vi "Teleop.vi"(10 "Match Info":T1={"Autonomous Elapsed Seconds"=0.0, "TeleOp Elapsed Seconds"=0.0, "Disabled Elapsed Seconds"=0.0, "Visited Autonomous"=FALSE, "Visited TeleOp"=FALSE, "Visited Disabled"=FALSE, "Autonomous Settings"={"Autonomous Style"=enum."Independent", "VI Refnum"=refnum}}, 11 "Call Context":T2) -> ()   [LabVIEW 2015]
doc: "This VI is called for each TeleOp packet received from the DS where the robot is not disabled. It is often used to read from the joysticks and update I/O or to update setpoints for timed control loops. It should complete and return within 20 milliseconds or it may miss DS packets."
uses:
  <vilib>/Rock Robotics/WPI/DriverStation/WPI_DriverStationDerivedRobotMode.ctl
  <vilib>/Rock Robotics/WPI/DriverStation/WPI_DriverStationMatch Info.ctl
  Common/Change Detect.vi
  Common/Change Detect Boolean.vi
  <vilib>/Rock Robotics/Network Tables/NT Read Boolean.vi
  <vilib>/Rock Robotics/Network Tables/NT Read Number.vi
  Robot Global Data.vi
  <vilib>/Rock Robotics/WPI/Utilities/WPI_GetSetVariantRefNum.vi
panel:
  out "Sample Slider 0":dbl(slide) scale=0.0..5.0
  out "Sample Boolean 1":bool
  out "Sample Boolean 0":bool
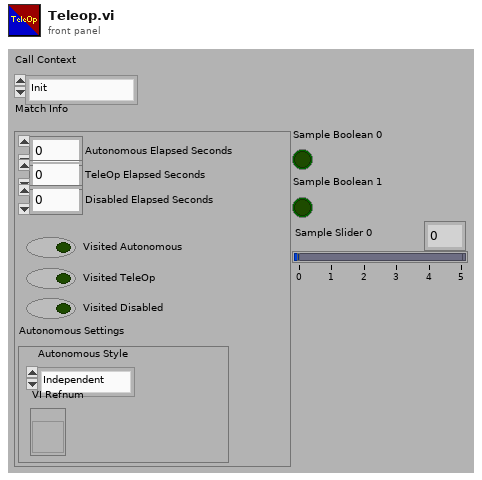
[diagram p1: front panel]
types:
  T1 = typedef "WPI_DriverStationMatch Info.ctl" = cluster{"Autonomous Elapsed Seconds":dbl, "TeleOp Elapsed Seconds":dbl, "Disabled Elapsed Seconds":dbl, "Visited Autonomous":bool, "Visited TeleOp":bool, "Visited Disabled":bool, "Autonomous Settings":cluster{"Autonomous Style":enum16{"Iterative", "Independent"}, "VI Refnum":refnum<vi>}}
  T2 = typedef "WPI_DriverStationDerivedRobotMode.ctl" = enum16{"Init", "Execute", "Stop"}
  T3 = typedef "WPI_DriverStationRobotMode2.ctl" = enum16{"Autonomous Disabled", "Autonomous Enabled", "Teleop Disabled", "Teleop Enabled", "Disconnected", "Finish", "Test Disabled", "Test Enabled", "Emergency Stopped"}
  T4 = typedef "WPI_JoystickDevRef.ctl" = cluster{"Device":T5}
  T5 = typedef "WPI_JoystickDeviceEnum.ctl" = enum16{"USB 0", "USB 1", "USB 2", "USB 3", "USB 4", "USB 5"}
  T6 = cluster{"Axes[0]":dbl, "Axes[1]":dbl, "Axes[2]":dbl, "Axes[3]":dbl, "Axes[4]":dbl, "Axes[5]":dbl, "Axes[6]":dbl, "Axes[7]":dbl, "Axes[8]":dbl}
  T7 = cluster{"Buttons[0]":bool, "Buttons[1]":bool, "Buttons[2]":bool, "Buttons[3]":bool, "Buttons[4]":bool, "Buttons[5]":bool, "Buttons[6]":bool, "Buttons[7]":bool, "Buttons[8]":bool}
  T8 = cluster{"Left_Trigger":dbl, "Right_Trigger ":dbl, "Left_X":dbl, "Left_Y":dbl, "Right_X":dbl, "Right_Y":dbl}
  T9 = cluster{"A":bool, "B":bool, "X":bool, " Y":bool, "LB":bool, " RB":bool, "Left_Thumb_Button":bool, "Right_Thumb_Button":bool, "Back":bool, "Start":bool}
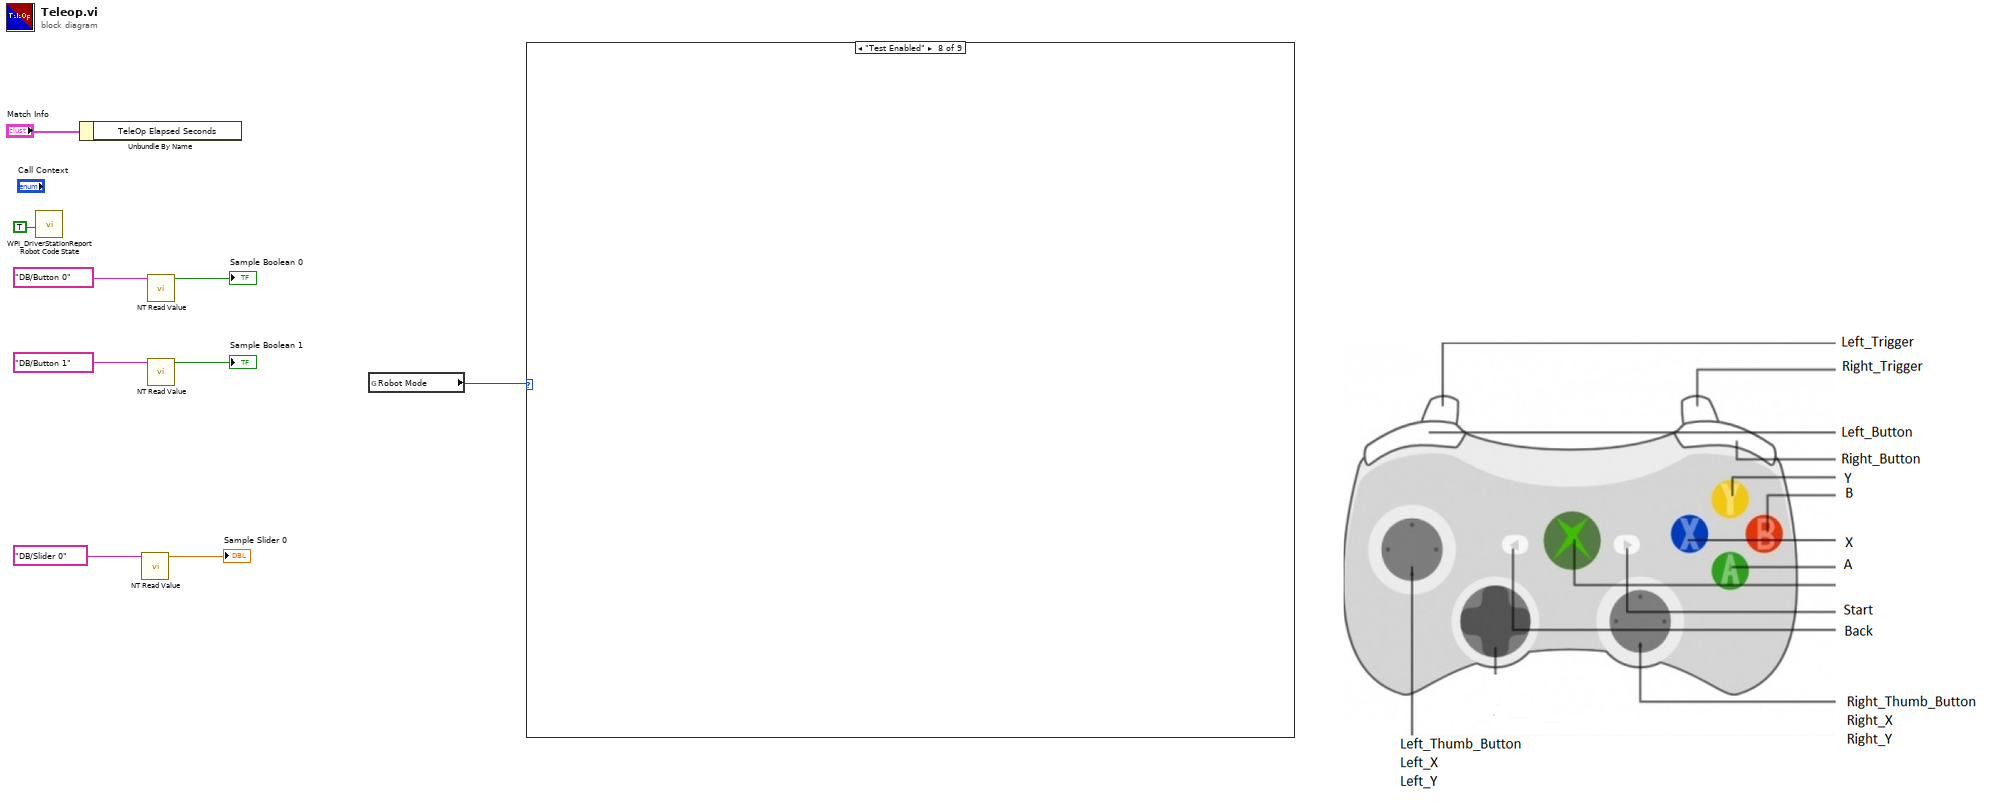
[diagram p0: block diagram]
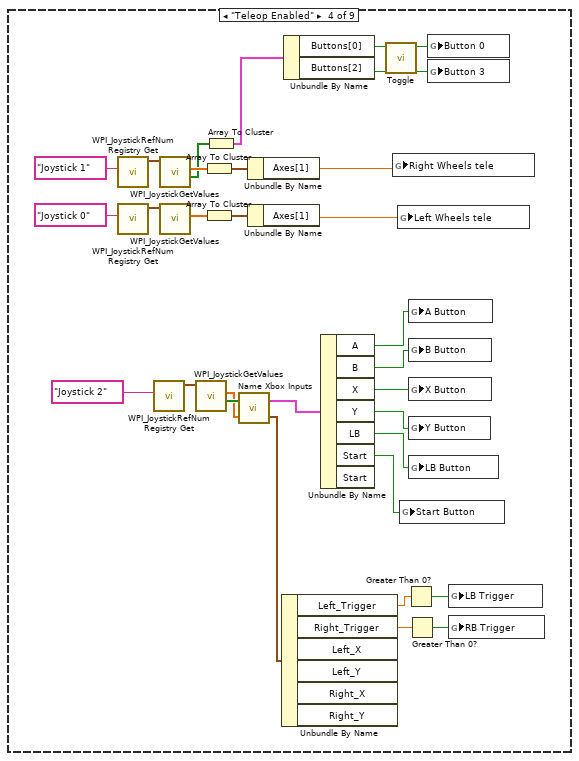
[diagram p5: hidden frame]
diagram:
  n1 = call <vilib>:"WPI_DriverStationReport Robot Code State.vi"("TeleOp"=TRUE ("Autonomous")) -> ()  [unwired: 10 in, 1 out]
  n2 = Unbundle By Name("Match Info") -> ()  [unwired: 1 out]
  n3 = call-poly <vilib>:"NT Read Value.vi"("Name"="DB/Slider 0" ("refnum name")) -> ("Numeric"=→"Sample Slider 0":dbl)  [unwired: 9 in, 1 out]
  n4 = call-poly <vilib>:"NT Read Value.vi"("Name"="DB/Button 0" ("refnum name")) -> ("Boolean"=→"Sample Boolean 0":bool)  [unwired: 9 in, 1 out]
  n5 = call-poly <vilib>:"NT Read Value.vi"("Name"="DB/Button 1" ("refnum name")) -> ("Boolean"=→"Sample Boolean 1":bool)  [unwired: 9 in, 1 out]
  n6 = global read "Robot Global Data.vi" "Robot Mode"() -> (w1:T3)
  n7 = case shown="\"Test Enabled\"" w1 {
    frame "Autonomous Disabled", Default {
    }
    frame "Autonomous Enabled" {
    }
    frame "Teleop Disabled" {
    }
    frame "Teleop Enabled" {
      n8 = call <vilib>:"WPI_JoystickRefNum Registry Get.vi"("refnum name"="Joystick 1") -> ("JoystickDevRef"=w38:T4)  [unwired: 1 in, 9 out]
      n9 = call <vilib>:"WPI_JoystickRefNum Registry Get.vi"("refnum name"="Joystick 0") -> ("JoystickDevRef"=w39:T4)  [unwired: 1 in, 9 out]
      n10 = call <vilib>:"WPI_JoystickRefNum Registry Get.vi"("refnum name"="Joystick 2") -> ("JoystickDevRef"=w31:T4)  [unwired: 1 in, 9 out]
      n11 = call <vilib>:"WPI_JoystickGetValues.vi"("JoystickDevRef"=w38) -> ("Buttons"=w19:bool[], "Axes"=w33:dbl[])  [unwired: 6 in, 3 out]
      n12 = call <vilib>:"WPI_JoystickGetValues.vi"("JoystickDevRef"=w39) -> ("Axes"=w36:dbl[])  [unwired: 6 in, 4 out]
      n13 = call <vilib>:"WPI_JoystickGetValues.vi"("JoystickDevRef"=w31) -> ("Buttons"=w30:bool[], "Axes"=w29:dbl[])  [unwired: 6 in, 3 out]
      n14 = Array To Cluster(array=w33) -> (cluster=w34:T6)
      n15 = Array To Cluster(array=w36) -> (cluster=w35:T6)
      n16 = Array To Cluster(array=w19) -> (cluster=w18:T7)
      n17 = call "Name Xbox Inputs.vi"("Axes"=w29, "Buttons"=w30) -> ("Named_Joystick"=w27:T8, "Named_Buttons"=w28:T9)
      n18 = Unbundle By Name(w34) -> ("Axes[1]"=w13:dbl)
      n19 = Unbundle By Name(w35) -> ("Axes[1]"=w14:dbl)
      n20 = Unbundle By Name(w27) -> ("Left_Trigger"=w10:dbl, "Right_Trigger"=w24:dbl)  [unwired: 4 out]
      n21 = Unbundle By Name(w18) -> ("Buttons[0]"=w17:bool, "Buttons[2]"=w12:bool)
      n22 = Unbundle By Name(w28) -> ("A"=w22:bool, "B"=w20:bool, "X"=w21:bool, "Y"=w26:bool, "LB"=w25:bool, "Start"=w15:bool)  [unwired: 1 out]
      n23 = call "Toggle.vi"("In"=w17) -> ("Toggled"=w16:bool)  [unwired: 10 in]
      n24 = global write "Robot Global Data.vi" "Right Wheels tele"(w13) -> ()
      n25 = global write "Robot Global Data.vi" "Left Wheels tele"(w14) -> ()
      n26 = global write "Robot Global Data.vi" "Start Button"(w15) -> ()
      n27 = Greater Than 0?(x=w10) -> (x > 0?=w11:bool)
      n28 = Greater Than 0?(x=w24) -> (x > 0?=w23:bool)
      n29 = global write "Robot Global Data.vi" "A Button"(w22) -> ()
      n30 = global write "Robot Global Data.vi" "B Button"(w20) -> ()
      n31 = global write "Robot Global Data.vi" "X Button"(w21) -> ()
      n32 = global write "Robot Global Data.vi" "Y Button"(w26) -> ()
      n33 = global write "Robot Global Data.vi" "LB Button"(w25) -> ()
      n34 = global write "Robot Global Data.vi" "Button 0"(w16) -> ()
      n35 = global write "Robot Global Data.vi" "Button 3"(w12) -> ()
      n36 = global write "Robot Global Data.vi" "LB Trigger"(w11) -> ()
      n37 = global write "Robot Global Data.vi" "RB Trigger"(w23) -> ()
    }
    frame "Disconnected" {
    }
    frame "Finish" {
    }
    frame "Test Disabled" {
    }
    frame "Test Enabled" {
    }
    frame "Emergency Stopped" {
    }
  }
